vi "Tokenize Value Response.vi"(8 "error in (no error)":errorcluster, 10 "Input":string, 11 "Tovey 9150 in":refnum<class "Tovey 9150.lvclass">) -> (0 "error out":errorcluster, 2 "Tokens":string[](array[string]), 3 "Tovey 9150 out":refnum<class "Tovey 9150.lvclass">)   [LabVIEW 2015, in "Tovey 9150.lvclass"]
uses:
  Tovey 9150.lvclass
  <userlib>/Common/ILC/ILCModelTypedefs/FinalDelimiter.ctl
  <userlib>/Common/ILC/ILCModelTypedefs/ILCModelTypedefs.lvlib
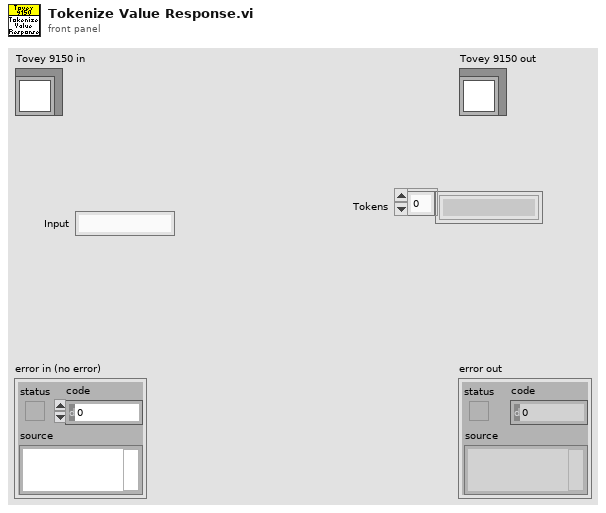
[diagram p1: front panel]
types:
  T1 = typedef "ILCCommon.lvlib/ILCModelTypedefs.lvlib/FinalDelimiter.ctl" = enum16{",", "<CR><LF>"}
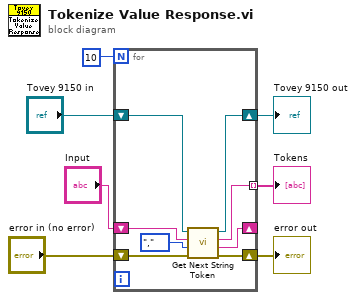
[diagram p0: block diagram]
diagram:
  n1 = for {
    N: 10 -> [_]
    shift-right: [w12] -> w6
    shift-left: "Tovey 9150 in" -> [w14]
    shift-right: [w11] -> _
    shift-left: "Input" -> [w15]
    tunnel: [w10] -> w2 mode=indexing
    shift-right: [w8] -> w4
    shift-left: "error in (no error)" -> [w9]
    n2 = call "Get Next String Token.vi"("error in (no error)"=w9, "Final Delimiter"=FinalDelimiter.",", "inputString"=w15, "TEI9150 in"=w14) -> ("error out"=w8:errorcluster, "remainingString"=w11:string, "extractedSegment"=w10:string, "TEI9150 out"=w12:refnum<class "Tovey 9150.lvclass">)  [unwired: 4 in]
  }
  "error out" <- w4
  "Tovey 9150 out" <- w6
  "Tokens" <- w2
